vi "448Issue.vi"() -> ()   [LabVIEW 2017]
uses:
  user.lib/_NEVSTOP/Communicable State Machine(CSM)/_Support/Typedef/_CSM_GlobalLog_MSG.ctl
  user.lib/_NEVSTOP/Communicable State Machine(CSM)/_Support/Typedef/_CSM_Response Source Message.ctl
  user.lib/_NEVSTOP/Communicable State Machine(CSM)/_Support/Typedef/_CSM_GlobalLog_MSG_TYPE.ctl
  user.lib/_NEVSTOP/Communicable State Machine(CSM)/Communicable State Machine.lvlib
  user.lib/_NEVSTOP/Communicable State Machine(CSM)/addons/Watchdog/CSM Watchdog.lvlib
panel:
  in  "Exit":bool
  out "State History":string
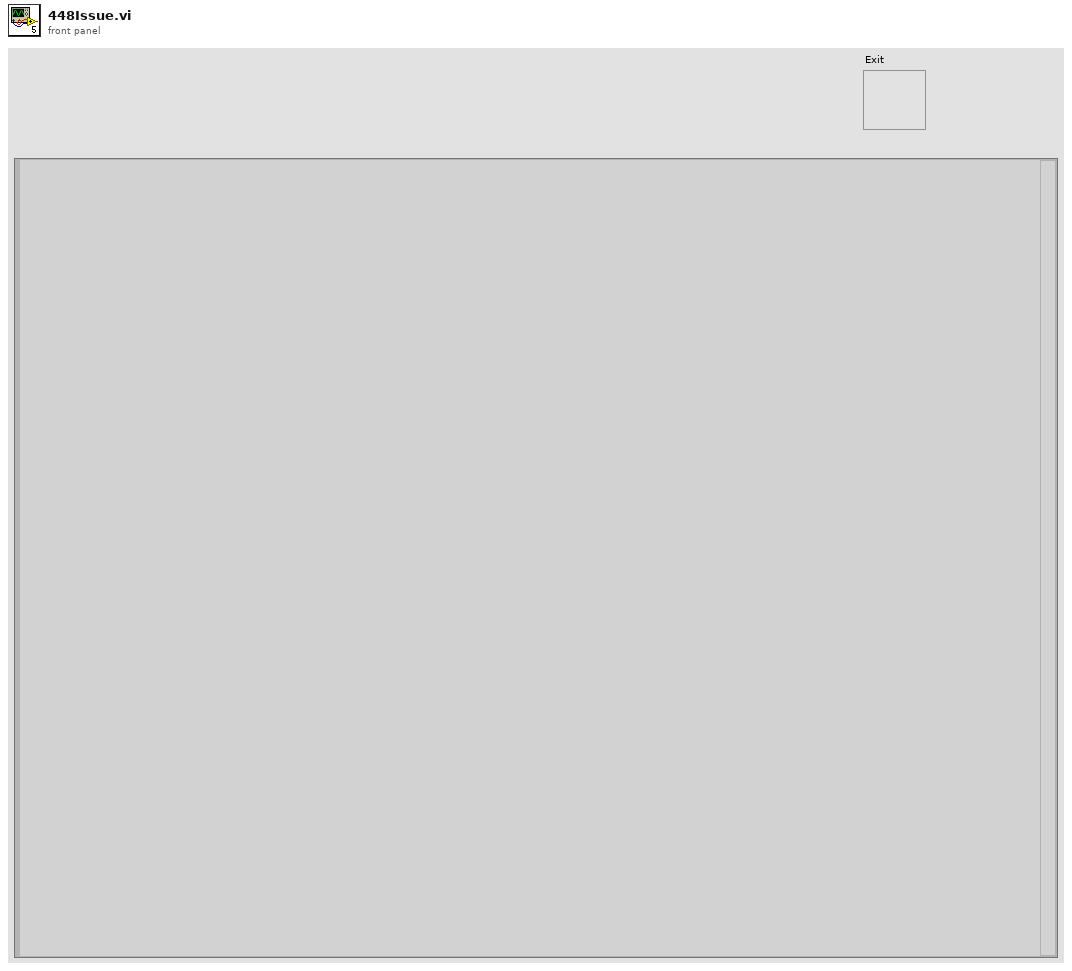
[diagram p1: front panel]
types:
  T1 = cluster{"threashold(#/s)":dbl, "Check Peroid(s)":dbl}
  T2 = typedef "Communicable State Machine.lvlib/_CSM_GlobalLog_MSG.ctl" = cluster{"Name(\"\" to use uuid)":string, "Current State":string, "Arguments":string, "Source Message":T3, "Source Module":string, "Complete(T)/Start(F)":bool, "LogType":T4}
  T3 = typedef "Communicable State Machine.lvlib/_CSM_Response Source Message.ctl" = cluster{"‘State":string, "’Arguments":string, "’Error":errorcluster}
  T4 = typedef "Communicable State Machine.lvlib/_CSM_GlobalLog_MSG_TYPE.ctl" = enum16{"User Log", "State Change", "Status", "Interrupt", "Register", "Unregister", "Error Log", "Module Created", "Module Destroyed"}
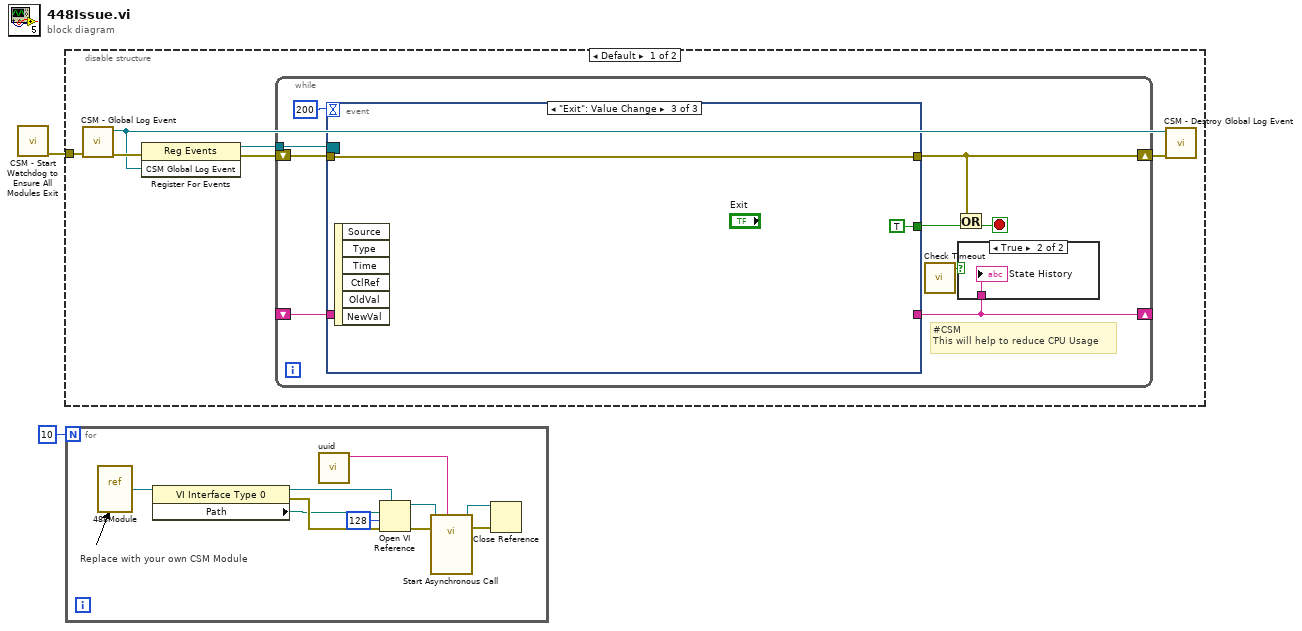
[diagram p0: block diagram]
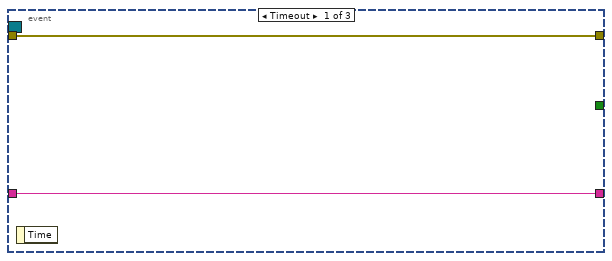
[diagram p3: hidden frame]
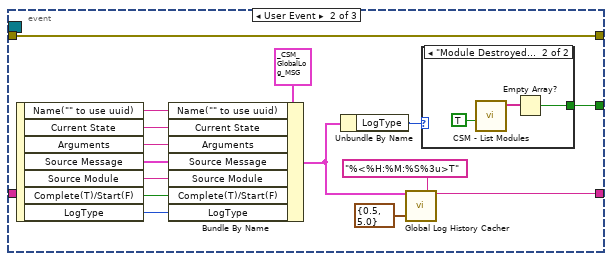
[diagram p4: hidden frame]
diagram:
  n1 = call "CSM - Start Watchdog to Ensure All Modules Exit.vi"() -> ("error out"=w2:errorcluster)  [unwired: 11 in]
  n2 = disable-structure shown="Default" {
    disable-tunnel: w2 -> [w3 _]
    frame condition #0 (active) {
      n3 = call "CSM - Global Log Event.vi"("Error in"=w3) -> ("Error out"=w6:errorcluster, "CSM Global Log Event"=w4:refnum<user-event>)  [unwired: 9 in]
      n4 = register-events(error in=w6, w4) -> (reference out=w7:refnum<event-registration>, error out=w8:errorcluster)  [unwired: 1 in]
      n5 = while {
        tunnel: w7 -> [w17]
        shift-right: [w14] -> w5
        shift-left: w8 -> [w16]
        shift-right: [w11] -> _
        shift-left: _ -> [w10]
        stop <- w15 stop-if-true
        # "#CSM\nThis will help to reduce CPU Usage"
        n6 = event shown="[2] \"Exit\": Value Change" {
          selector: w17 -> [_ _ _]
          dyn-events: _ -> [_ _ _]
          timeout: 200 -> [_ _ _]
          tunnel: w16 -> [w20 w35 w40]
          tunnel: [w20 w35 w40] -> w14
          tunnel: [_ w24 TRUE ("empty?")] -> w13
          tunnel: [w19 w21 _] -> w11
          tunnel: w10 -> [w19 _ _]
          event Timeout {
            n7 = event-data() -> ()  [unwired: 1 in, 1 out]
          }
          event User Event {
            n8 = event-data() -> ("Name(\"\" to use uuid)"=w34:string, "Current State"=w33:string, "Arguments"=w32:string, "Source Message"=w31:T3, "Source Module"=w30:string, "Complete(T)/Start(F)"=w29:bool, "LogType"=w28:T4)  [unwired: 1 in]
            n9 = Bundle By Name(cluster=T2 {"Name(\"\" to use uuid)"="", "Current State"="", "Arguments"="", "Source Message"={"‘State"="", "’Arguments"="", "’Error"={"status"=FALSE, "code"=0, "source"=""}}, "Source Module"="", "Complete(T)/Start(F)"=FALSE, "LogType"=enum."State Change"} ("Cross CSM Data"), "Name(\"\" to use uuid)"=w34, "Current State"=w33, "Arguments"=w32, "Source Message"=w31, "Source Module"=w30, "Complete(T)/Start(F)"=w29, "LogType"=w28) -> (w26:T2)
            n10 = Unbundle By Name(w26) -> ("LogType"=w25:T4)
            n11 = call "Global Log History Cacher.vi"("Cross CSM Data"=w26, "Time format string"="%<%H:%M:%S%3u>T", "Settings"=T1 {"threashold(#/s)"=0.5, "Check Peroid(s)"=5.0}) -> ("String Cache"=w21:string)  [unwired: 11 in, 1 out]
            n12 = case shown="\"Module Destroyed\"" w25 {
              tunnel: [_ w36] -> w24
              frame "User Log", Default {
              }
              frame "Module Destroyed" {
                n13 = call "CSM - List Modules.vi"("With Instance(F)"=TRUE ("All?")) -> ("Module Names"=w38:string[])  [unwired: 9 in, 1 out]
                n14 = Empty Array?(array=w38) -> (empty?=w36:bool)
              }
            }
          }
          event "Exit": Value Change {
            n15 = event-data() -> ()  [unwired: 1 in, 6 out]
          }
        }
        n16 = call "Check Timeout.vi"() -> ("Timeout"=w9:bool)  [unwired: 8 in]
        n17 = Or(x=w14, y=w13) -> (x .or. y?=w15:bool)
        n18 = case shown="True" w9 {
          tunnel: w11 -> [_ w18]
          frame False {
          }
          frame True {
            "State History" <- w18
          }
        }
      }
      n19 = call "CSM - Destroy Global Log Event.vi"("Error in"=w5, "CSM Global Log Event"=w4) -> ()  [unwired: 9 in, 1 out]
    }
    frame condition #1 {
    }
  }
  n20 = for {
    N: 10 -> [_]
    # "Replace with your own CSM Module"
    n21 = vi-ref "488Module.vi"() -> (w43:refnum<vi>)
    n22 = property class="VI Interface Type 0"(reference=w43) -> (reference out=w47:refnum<vi>, error out=w45:errorcluster, "Path"=w44:path)  [unwired: 1 in]
    n23 = call "uuid.vi"() -> ("UUID"=w41:string)  [unwired: 11 in]
    n24 = Open VI Reference(type specifier VI Refnum (for type only)=w47, vi path=w44, options=128, error in (no error)=w45) -> (vi reference=w46:refnum<vi>, error out=w42:errorcluster)  [unwired: 2 in]
    n25 = call-by-ref "Start Asynchronous Call"(reference=w46, error in=w42, "Name(\"\" to use uuid)"=w41) -> (reference out=w49:refnum<vi>, error out=w48:errorcluster)  [unwired: 11 in]
    n26 = Close Reference(reference=w49, error in (no error)=w48) -> ()  [unwired: 1 out]
  }
